vi "changeTimeScale.vi"(8 "error in (no error)":errorcluster, 10 "timescale":dbl, 11 "AnalysisResultsViewer in":refnum<class "AnalysisResultsViewer.lvclass">) -> (0 "error out":errorcluster, 3 "AnalysisResultsViewer out":refnum<class "AnalysisResultsViewer.lvclass">)   [LabVIEW 2009, in "Views.lvlib" / "Camera.lvlib" / "AnalysisResultsViewer.lvclass"]
uses:
  AnalysisResultsViewer.lvclass
  AnalysisResultsViewer.lvclass/AnalysisResultsViewer.ctl
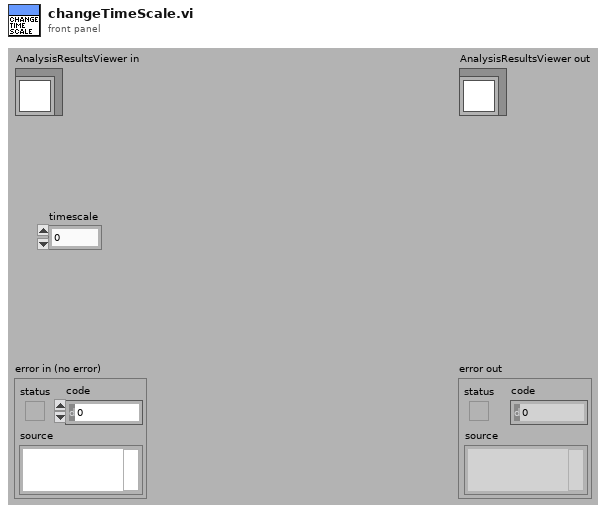
[diagram p1: front panel]
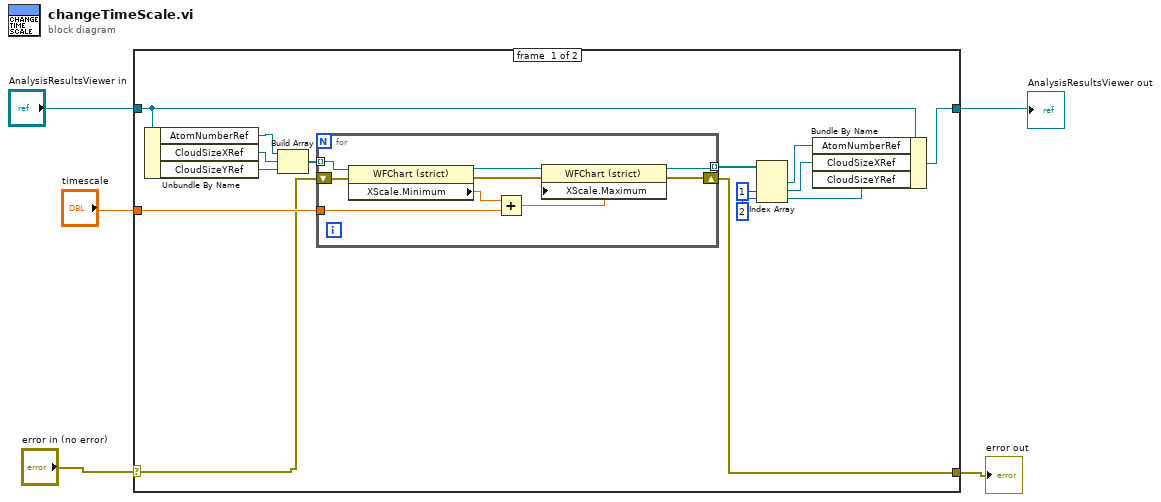
[diagram p0: block diagram]
diagram:
  n1 = case shown="No Error" "error in (no error)" {
    selector: "error in (no error)" -> [w15 w31]
    tunnel: [w14 w31] -> w4
    tunnel: [w6 w30] -> w2
    tunnel: "AnalysisResultsViewer in" -> [w7 w30]
    tunnel: "timescale" -> [w20 _]
    frame #0 {
      n2 = Unbundle By Name(w7) -> ("AtomNumberRef"=w17:refnum<vi>, "CloudSizeXRef"=w18:refnum<vi>, "CloudSizeYRef"=w19:refnum<vi>)
      n3 = Build Array(w17, w18, w19) -> (w16:refnum<vi>[])
      n4 = for {
        tunnel: w20 -> [w26]
        tunnel: w16 -> [w24] mode=indexing
        shift-right: [w21] -> w14
        shift-left: w15 -> [w23]
        tunnel: [w22] -> w13 mode=indexing
        n5 = property class="WFChart (strict)"(reference=w24, error in=w23) -> (reference out=w29:refnum<vi>, error out=w28:errorcluster, "XScale.Minimum"=w27:dbl)
        n6 = Add(x=w27, y=w26) -> (x+y=w25:dbl)
        n7 = property class="WFChart (strict)"(reference=w29, error in=w28, "XScale.Maximum"=w25) -> (reference out=w22:refnum<vi>, error out=w21:errorcluster)
      }
      n8 = Index Array(array=w13, index #2=1, index #3=2) -> (element #1=w8:refnum<vi>, element #2=w9:refnum<vi>, element #3=w10:refnum<vi>)  [unwired: 1 in]
      n9 = Bundle By Name(cluster=w7, "AtomNumberRef"=w8, "CloudSizeXRef"=w9, "CloudSizeYRef"=w10) -> (w6:refnum<class "AnalysisResultsViewer.lvclass">)
    }
    frame #1 {
    }
  }
  "error out" <- w4
  "AnalysisResultsViewer out" <- w2
